vi "Read Atts.vi"(8 "error in (no error)":errorcluster, 11 "RS in":refnum<class "RS.lvclass">) -> (0 "error out":errorcluster, 1 "IF_Band":dbl, 2 "Stop":dbl, 3 "RS out":refnum<class "RS.lvclass">, 4 "Points":i32, 5 "Start":dbl)   [LabVIEW 2015, in "RS.lvclass"]
uses:
  RS.lvclass
  RS.lvclass/RS.ctl
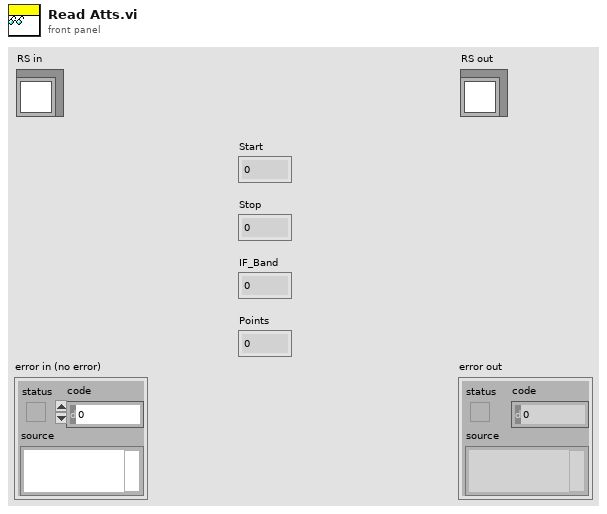
[diagram p1: front panel]
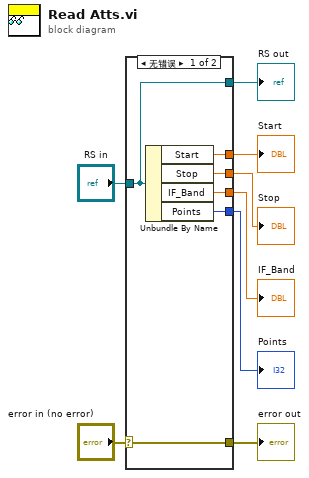
[diagram p0: block diagram]
diagram:
  n1 = case shown="无错误" "error in (no error)" {
    selector: "error in (no error)" -> [w14 w16]
    tunnel: [w14 w16] -> w2
    tunnel: [w13 _] -> w6
    tunnel: [w12 _] -> w5
    tunnel: [w11 _] -> w4
    tunnel: [w10 _] -> w1
    tunnel: "RS in" -> [w9 w15]
    tunnel: [w9 w15] -> w7
    frame No Error {
      n2 = Unbundle By Name(w9) -> ("Start"=w13:dbl, "Stop"=w12:dbl, "IF_Band"=w11:dbl, "Points"=w10:i32)
    }
    frame Error {
    }
  }
  "error out" <- w2
  "RS out" <- w7
  "Stop" <- w5
  "IF_Band" <- w4
  "Points" <- w1
  "Start" <- w6
